vi "Parzen Window (DBL).vi"(11 "X":dbl[](array[numeric])) -> (0 "error":i32, 3 "Windowed X":dbl[](array[numeric]))   [LabVIEW 2017, in "NI_AALPro.lvlib"]
doc: "Applies a Parzen window to the input signal <B>X</B>. Wire data to the <B>X</B> input to determine the polymorphic instance to use or manually select the instance."
uses:
  NI_AALPro.lvlib
  <resource>/lvanlys.dll
panel:
  # "Parzen Window"
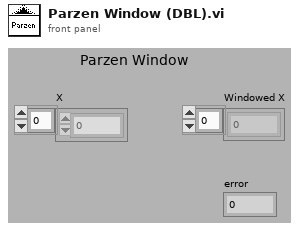
[diagram p1: front panel]
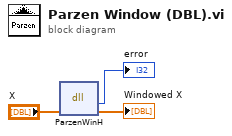
[diagram p0: block diagram]
diagram:
  n1 = dll-call lib="C:/Program Files (x86)/National Instruments/LabVIEW 2017/resource/lvanlys.*" fn="ParzenWinH"("X"="X") -> ("error"=→"error":i32, "X"=→"Windowed X":dbl[])  [unwired: 3 in, 2 out]
